vi "Operations Monitor.vi"() -> ()   [LabVIEW 2016, in "Top Level.lvlib"]
doc: "This VI is part of the Top Level library of VIs that are opened upon startup. Vacuum pressures are read via serial connections between the vacuum gauge controller and the nearest cRIO. At the cRIO, a Real-Time VI puts the pressures into shared variables which are displayed here. \n\nThe individual cRIOs are pinged to check network connections and cRIO resources are from shared variables. \n\nThe Omega CNi854 Controller/Monitor measures temperature of Cs Oven on ion source and is communicated with directly over TCP."
uses:
  Top Level.lvlib
  <vilib>/Utility/miscctls.llb/LVRowAndColumnTypeDef.ctl
  cRIO code/SCA/controls/GP307 cluster.ctl
panel:
  in  "Tab Control":T1(tab)
  out "LE Waist":string
  out "Tank Entrance":string
  out "Tank Exit":string
  out "Analyzer Image":string
  out "HE Waist/Analyzer Object":string
  out "Transmission":string
  out "R30 Switch Image":string
  out "R30 Detector":string
  out "R30 ESA":string
  in  "stop":bool
  out "date/time string":string
  out "Injector A Image":string
  out "Injector A Object":string
  out "Terminal Voltage":dbl format="%#_4g"
  out "R45 EXB":string
  out "R45 Switch Image":string
  out "R45 Waist":string
  out "SCA bellows":string
  out "SCA source":string
  in  "Ping Timeout (ms)":i32=100
  out "cRIO Status":i32(listbox)
  out "Oven Temperature":dbl(graph)
  out "Oven Temp (°C)":dbl
  in  "Omega VISA resource":refnum<visa-resource-name>="TCPIP0::192.168.1.173::2000::SOCKET"
  out "Omega Iteration":i32
  in  "byte count":u32=15
  in  "Wait (ms)":u32=500
  out "Read errors":i32
  out "Omega read buffer":string
  out "SV read error":errorcluster
  out "Terminal read error":errorcluster
  out "Ping error":errorcluster
  in  "Clear Ping Error":bool
  out "cRIO SV error":errorcluster
  in  "Clear SV Error":bool
  out "Omega T error":errorcluster
  # "VACUUM  PRESSURES"
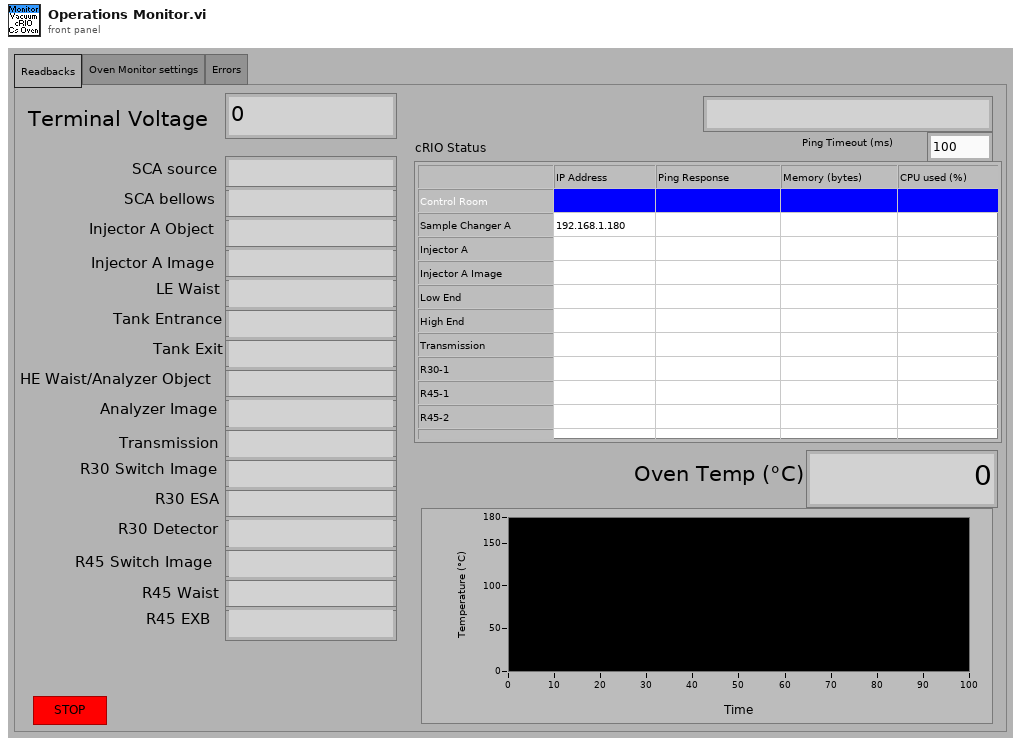
[diagram p1: front panel]
types:
  T1 = enum32{"Readbacks", "Oven Monitor settings", "Errors"}
  T2 = typedef "LVRowAndColumnTypeDef.ctl" = cluster{"Row":i32, "Column":i32}
  T3 = typedef "GP307 cluster.ctl" = cluster{"Ion gauge 1":string, "Convectron  Gauge 1 ":string, "Ion Gauge 2":string, "Convectrom Gauge 2":string}
  T4 = cluster{"Ion gauge 1":string, "Convectron  Gauge 1 ":string, "Ion Gauge 2":string, "Convectrom Gauge 2":string}
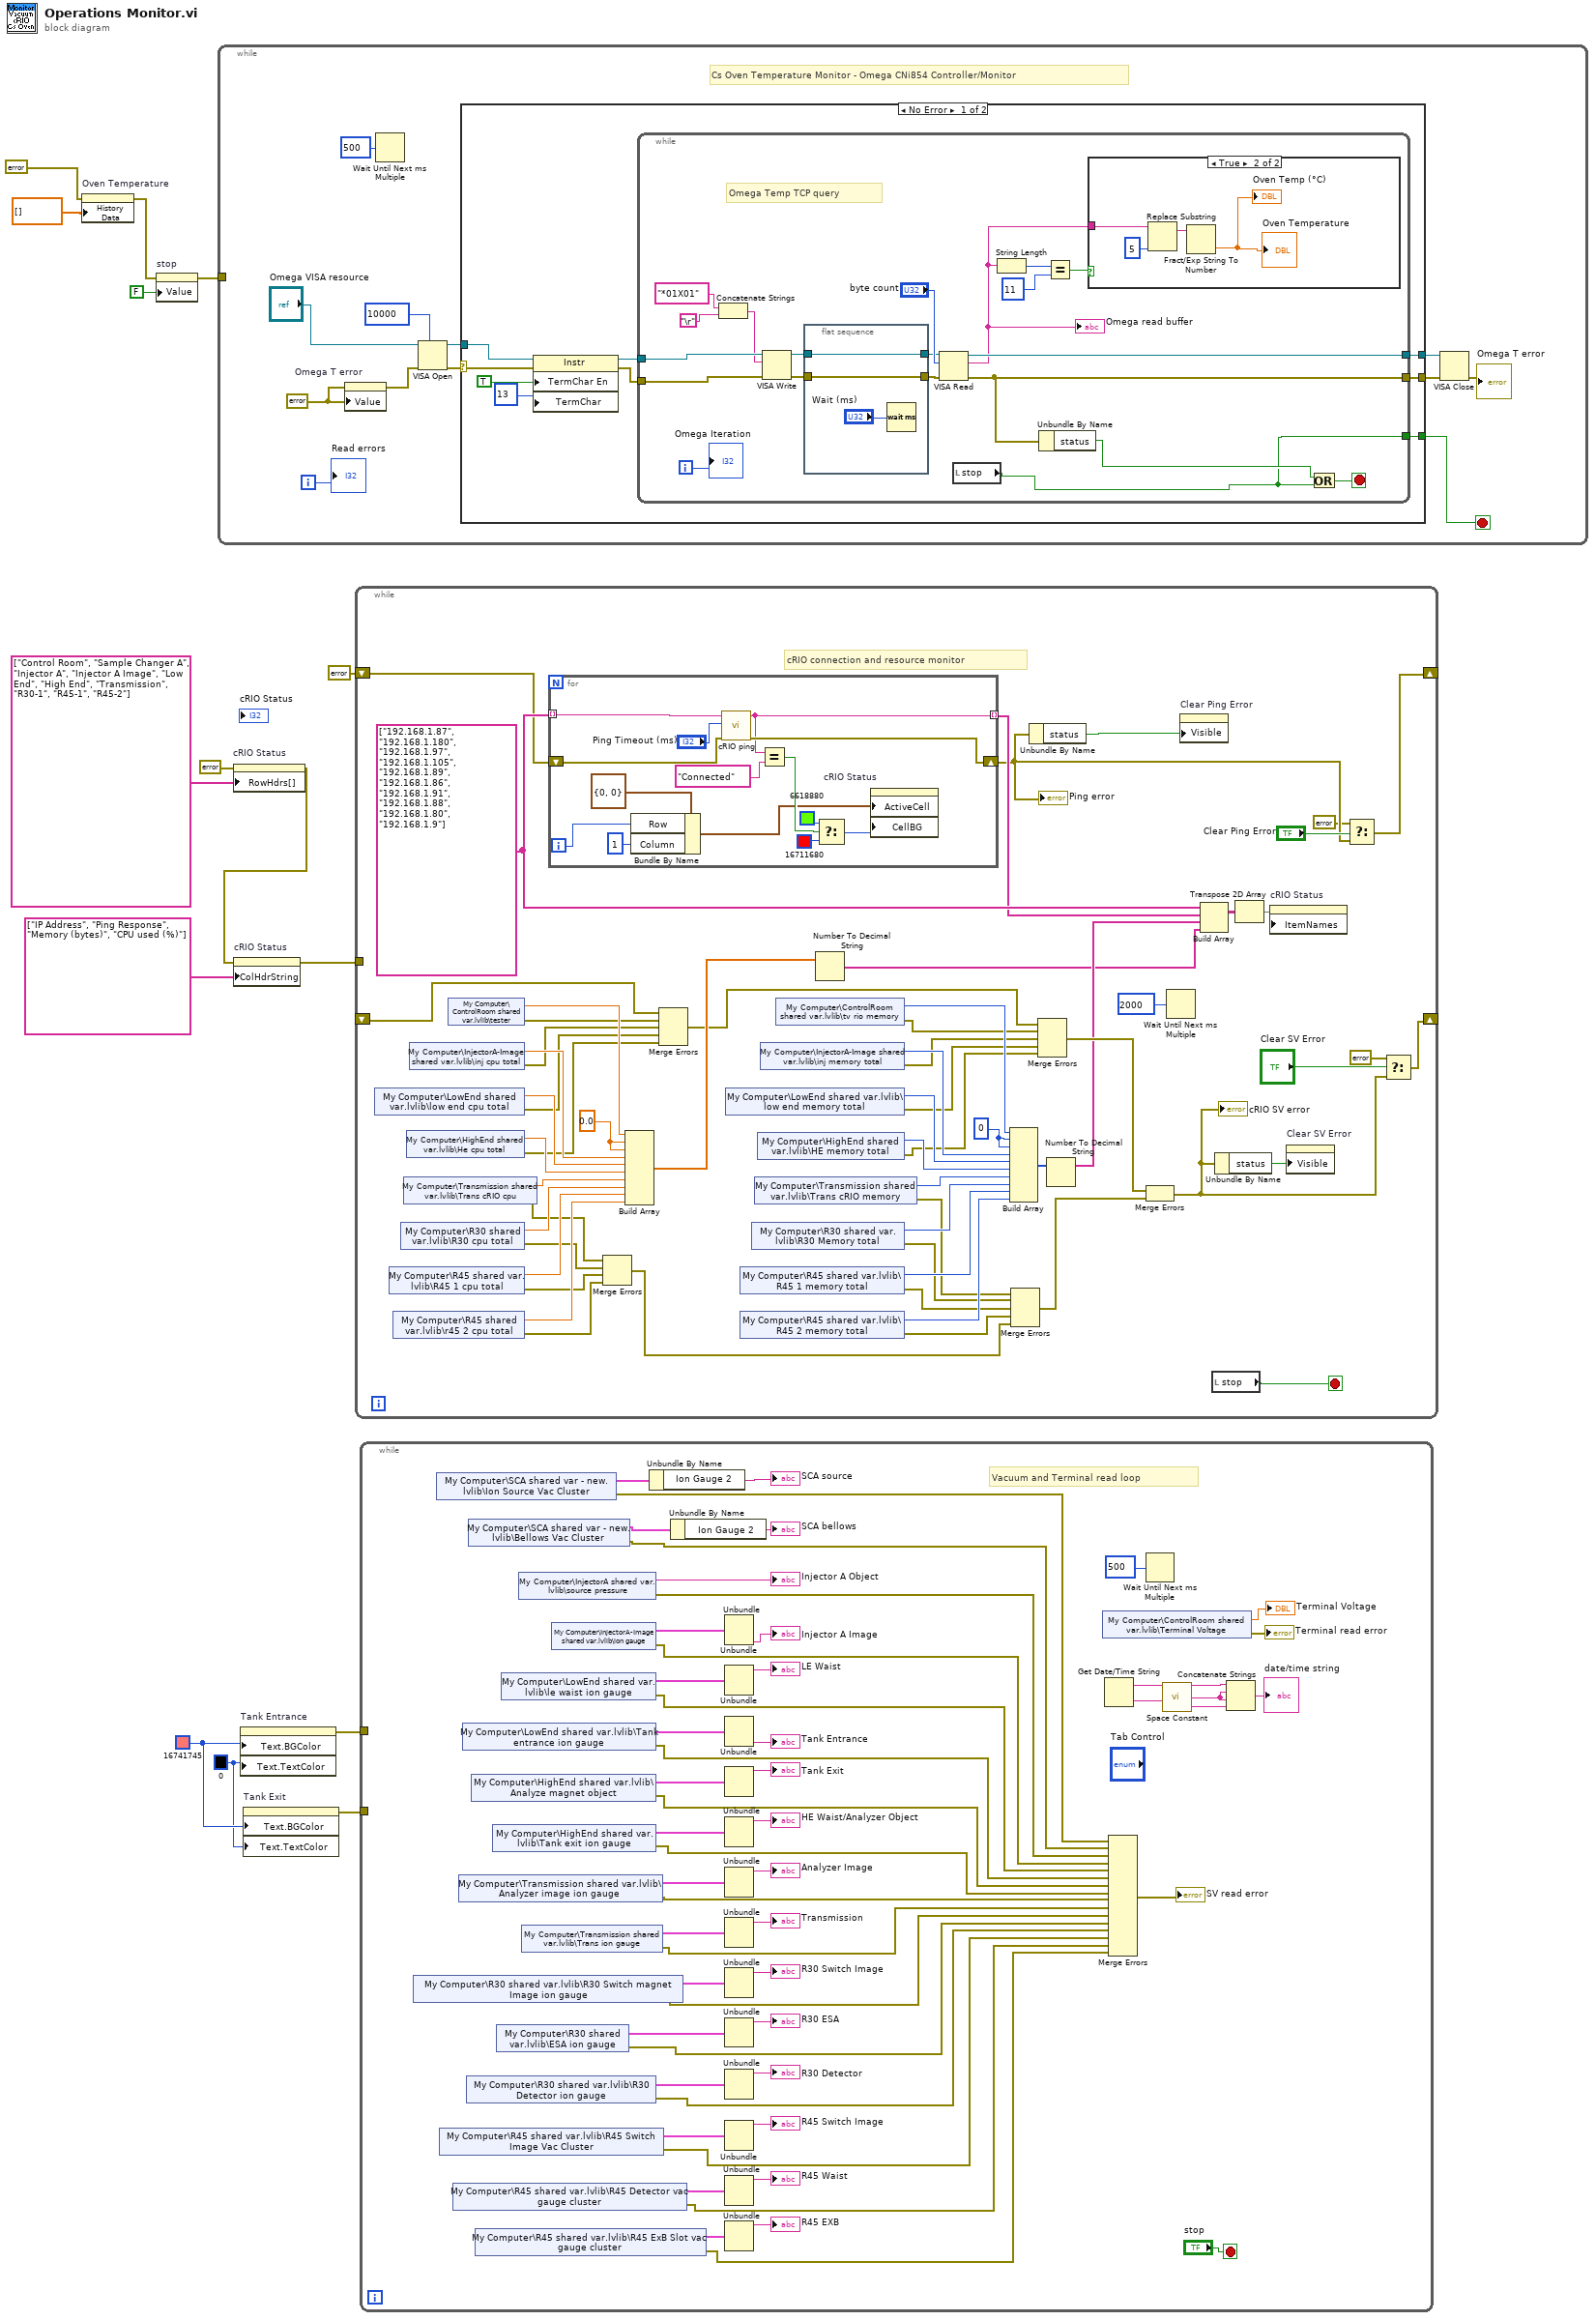
[diagram p0: block diagram]
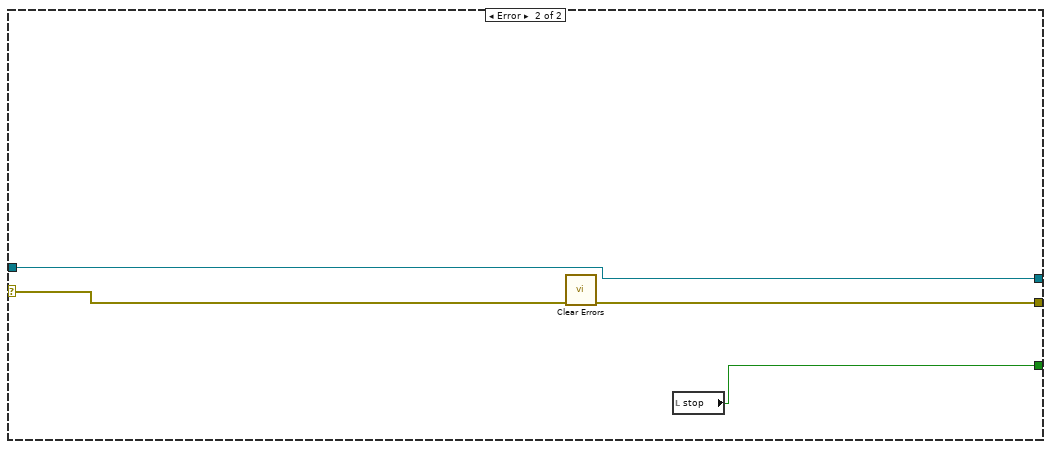
[diagram p3: hidden frame]
diagram:
  w1 = u32 0 ("Text.Text Colors:Text Color")
  w2 = u32 16741745 ("Text.Text Colors:BG Color")
  n1 = property on="Oven Temperature" class="WFChart (strict)"(error in=errorcluster {"status"=FALSE, "code"=0, "source"=""} ("error in (no error)"), "History Data"=dbl[] []) -> (error out=w6:errorcluster)  [unwired: 1 in, 1 out]
  n2 = property on="stop" class="Bool (strict)"(error in=w6, "Value"=FALSE ("stop")) -> (error out=w5:errorcluster)  [unwired: 1 in, 1 out]
  n3 = while {
    tunnel: w5 -> [_]
    i -> [w19]
    stop <- w20 stop-if-true
    w22 = errorcluster {"status"=FALSE, "code"=0, "source"=""} ("error in (no error)")
    # "Cs Oven Temperature Monitor - Omega CNi854 Controller/Monitor"
    # "Omega Temperature Monitor Loop"
    n4 = property on="Omega T error" class="Clust (strict)"(error in=w22, "Value"=w22) -> (error out=w23:errorcluster)  [unwired: 1 in, 1 out]
    n5 = Wait Until Next ms Multiple(millisecond multiple=u32 500) -> ()  [unwired: 1 out]
    n6 = VISA Open(timeout (0)=u32 10000 ("VISA Open timeout (0)"), error in (no error)=w23, VISA resource name="Omega VISA resource") -> (VISA resource name=w27:refnum<visa-resource-name>, error out=w18:errorcluster)  [unwired: 2 in]
    n7 = case shown="No Error" w18 {
      selector: w18 -> [w29 w66]
      tunnel: w27 -> [w34 w67]
      tunnel: [w36 w67] -> w26
      tunnel: [w35 w65] -> w25
      tunnel: [w30 w64] -> w20
      frame No Error {
        n8 = property class="Instr"(reference=w34, error in=w29, "TermChar En"=TRUE ("Message Based Settings:Termination Character Enable"), "TermChar"=u8 13 ("Message Based Settings:Termination Character")) -> (reference out=w33:refnum<visa-resource-name>, error out=w28:errorcluster)
        n9 = while {
          tunnel: w33 -> [w52]
          tunnel: [w56] -> w36
          tunnel: w28 -> [w47]
          tunnel: [w55] -> w35
          tunnel: [w37] -> w30
          i -> [w53]
          stop <- w54 stop-if-true
          # "Omega Temp TCP query"
          n10 = Concatenate Strings("*01X01" ("data in"), "\r") -> (w49:string)
          n11 = VISA Write(VISA resource name=w52, write buffer=w49, error in (no error)=w47) -> (VISA resource name out=w40:refnum<visa-resource-name>, error out=w42:errorcluster)  [unwired: 1 out]
          n12 = flat-sequence {
            tunnel: w42 -> [w59]
            tunnel: [w59] -> w41
            tunnel: w40 -> [w58]
            tunnel: [w58] -> w39
            frame #0 {
              n13 = Wait (ms)(milliseconds to wait="Wait (ms)") -> ()  [unwired: 1 out]
            }
          }
          n14 = VISA Read(VISA resource name=w39, byte count="byte count", error in (no error)=w41) -> (VISA resource name out=w56:refnum<visa-resource-name>, read buffer=w43:string, error out=w55:errorcluster)  [unwired: 1 out]
          "Omega read buffer" <- w43
          n15 = local read "stop"() -> (w37:bool)
          n16 = String Length(string=w43) -> (length=w46:i32)
          n17 = Unbundle By Name(w55) -> ("status"=w38:bool)
          n18 = Equal?(x=w46, y=11) -> (x = y?=w44:bool)
          n19 = case shown="True" w44 {
            tunnel: w43 -> [_ w60]
            frame False {
            }
            frame True {
              n20 = Replace Substring(2:5 ("length (len. of substring)"), 5:w60) -> (1:w61:string)  [unwired: 2 in, 1 out]
              n21 = Fract/Exp String To Number(string=w61) -> (number=→"Oven Temp (°C)" →"Oven Temperature":dbl)  [unwired: 3 in, 1 out]
            }
          }
          n22 = Or(x=w38, y=w37) -> (x .or. y?=w54:bool)
          "Omega Iteration" <- w53
        }
      }
      frame Error {
        n23 = call <vilib>:"Clear Errors.vi"("error in (no error)"=w66) -> ("error out"=w65:errorcluster)  [unwired: 5 in, 1 out]
        n24 = local read "stop"() -> (w64:bool)
      }
    }
    n25 = VISA Close(VISA resource name=w26, error in (no error)=w25) -> (error out=→"Omega T error":errorcluster)
    "Read errors" <- w19
  }
  n26 = property on="cRIO Status" class="MCListbox (strict)"(error in=errorcluster {"status"=FALSE, "code"=0, "source"=""} ("error out"), "RowHdrs[]"=string[] ["Control Room", "Sample Changer A", "Injector A", "Injector A Image", "Low End", "High End", "Transmission", "R30-1", "R45-1", "R45-2"]) -> (error out=w10:errorcluster)  [unwired: 1 in, 1 out]
  n27 = property on="cRIO Status" class="MCListbox (strict)"(error in=w10, "ColHdrString"=string[] ["IP Address", "Ping Response", "Memory (bytes)", "CPU used (%)"]) -> (error out=w13:errorcluster)  [unwired: 1 in, 1 out]
  n28 = property on="Tank Entrance" class="Str"("Text.BGColor"=w2, "Text.TextColor"=w1) -> (error out=w3:errorcluster)  [unwired: 2 in, 1 out]
  n29 = property on="Tank Exit" class="Str"("Text.BGColor"=w2, "Text.TextColor"=w1) -> (error out=w4:errorcluster)  [unwired: 2 in, 1 out]
  n30 = while {
    shift-right: [w72] -> _
    shift-left: _ -> [w97]
    shift-right: [w79] -> _
    shift-left: errorcluster {"status"=FALSE, "code"=0, "source"=""} ("Ping error out") -> [w104]
    tunnel: w13 -> [_]
    stop <- w70 stop-if-true
    w106 = string[] ["192.168.1.87", "192.168.1.180", "192.168.1.97", "192.168.1.105", "192.168.1.89", "192.168.1.86", "192.168.1.91", "192.168.1.88", "192.168.1.80", "192.168.1.9"]
    w107 = u32 0 ("element")
    w108 = 0.0 ("element")
    # "cRIO connection and resource monitor"
    n31 = shared-variable "My Computer\\LowEnd shared var.lvlib\\low end cpu total"() -> (w124:dbl, error out=w99:errorcluster)  [unwired: 1 in]
    n32 = shared-variable "My Computer\\R45 shared var.lvlib\\R45 1 cpu total"() -> (w120:dbl, error out=w96:errorcluster)  [unwired: 1 in]
    n33 = shared-variable "My Computer\\R45 shared var.lvlib\\r45 2 cpu total"() -> (w119:dbl, error out=w93:errorcluster)  [unwired: 1 in]
    n34 = shared-variable "My Computer\\R30 shared var.lvlib\\R30 cpu total"() -> (w121:dbl, error out=w95:errorcluster)  [unwired: 1 in]
    n35 = shared-variable "My Computer\\Transmission shared var.lvlib\\Trans cRIO cpu"() -> (w122:dbl, error out=w94:errorcluster)  [unwired: 1 in]
    n36 = shared-variable "My Computer\\HighEnd shared var.lvlib\\He cpu total"() -> (w123:dbl, error out=w98:errorcluster)  [unwired: 1 in]
    n37 = shared-variable "My Computer\\InjectorA-Image shared var.lvlib\\inj cpu total"() -> (w125:dbl, error out=w100:errorcluster)  [unwired: 1 in]
    n38 = shared-variable "My Computer\\ControlRoom shared var.lvlib\\tester"() -> (w126:dbl, error out=w101:errorcluster)  [unwired: 1 in]
    n39 = for {
      tunnel: w106 -> [w140] mode=indexing
      tunnel: [w137] -> w105 mode=indexing
      shift-right: [w138] -> w77
      shift-left: w104 -> [w139]
      i -> [w130]
      n40 = Bundle By Name(cluster=T2 {"Row"=0, "Column"=0} ("Active Cell:Active Cell"), "Row"=w130, "Column"=1) -> (w129:T2)
      n41 = call "cRIO ping.vi"("Error in"=w139, "Ping Timeout (ms)"="Ping Timeout (ms)", "IP Address"=w140) -> ("Ping error out"=w138:errorcluster, "Ping Response"=w137:string)  [unwired: 7 in]
      n42 = Equal?(x=w137, y="Connected" ("t")) -> (x = y?=w134:bool)
      n43 = Select(t=u32 6618880, s=w134, f=u32 16711680) -> (s? t:f=w135:u32)
      n44 = property on="cRIO Status" class="MCListbox (strict)"("ActiveCell"=w129, "CellBG"=w135) -> ()  [unwired: 2 in, 2 out]
    }
    "Ping error" <- w77
    n45 = Merge Errors(w94, w95, w96, w93) -> (w82:errorcluster)
    n46 = Build Array(w126, w108, w108, w125, w124, w123, w122, w121, w120, w119) -> (w109:dbl[])
    n47 = Merge Errors(w97, w101, w100, w99, w98) -> (w92:errorcluster)
    n48 = shared-variable "My Computer\\LowEnd shared var.lvlib\\low end memory total"() -> (w112:u32, error out=w89:errorcluster)  [unwired: 1 in]
    n49 = shared-variable "My Computer\\R45 shared var.lvlib\\R45 1 memory total"() -> (w116:u32, error out=w86:errorcluster)  [unwired: 1 in]
    n50 = shared-variable "My Computer\\R45 shared var.lvlib\\R45 2 memory total"() -> (w117:u32, error out=w87:errorcluster)  [unwired: 1 in]
    n51 = shared-variable "My Computer\\R30 shared var.lvlib\\R30 Memory total"() -> (w115:u32, error out=w85:errorcluster)  [unwired: 1 in]
    n52 = shared-variable "My Computer\\Transmission shared var.lvlib\\Trans cRIO memory"() -> (w114:u32, error out=w84:errorcluster)  [unwired: 1 in]
    n53 = shared-variable "My Computer\\HighEnd shared var.lvlib\\HE memory total"() -> (w111:u32, error out=w88:errorcluster)  [unwired: 1 in]
    n54 = shared-variable "My Computer\\InjectorA-Image shared var.lvlib\\inj memory total"() -> (w113:u32, error out=w90:errorcluster)  [unwired: 1 in]
    n55 = shared-variable "My Computer\\ControlRoom shared var.lvlib\\tv rio memory"() -> (w118:u32, error out=w91:errorcluster)  [unwired: 1 in]
    n56 = Number To Decimal String(number=w109) -> (decimal integer string=w68:string[])  [unwired: 1 in]
    n57 = Build Array(w118, w107, w107, w113, w112, w111, w114, w115, w116, w117) -> (w110:u32[])
    n58 = Merge Errors(w84, w85, w86, w87, w82) -> (w83:errorcluster)
    n59 = Unbundle By Name(w77) -> ("status"=w80:bool)
    n60 = Merge Errors(w92, w91, w90, w89, w88) -> (w81:errorcluster)
    n61 = Number To Decimal String(number=w110) -> (decimal integer string=w69:string[])  [unwired: 1 in]
    n62 = Merge Errors(w81, w83) -> (w71:errorcluster)
    "cRIO SV error" <- w71
    n63 = Wait Until Next ms Multiple(millisecond multiple=u32 2000) -> ()  [unwired: 1 out]
    n64 = property on="Clear Ping Error" class="Bool"("Visible"=w80) -> ()  [unwired: 2 in, 2 out]
    n65 = Build Array(w106, w105, w69, w68) -> (w103:string[][])
    n66 = local read "stop"() -> (w70:bool)
    n67 = Unbundle By Name(w71) -> ("status"=w75:bool)
    n68 = Transpose 2D Array(2D array=w103) -> (transposed array=w102:string[][])
    n69 = property on="cRIO Status" class="MCListbox (strict)"("ItemNames"=w102) -> ()  [unwired: 2 in, 2 out]
    n70 = property on="Clear SV Error" class="Bool"("Visible"=w75) -> ()  [unwired: 2 in, 2 out]
    n71 = Select(t=errorcluster {"status"=FALSE, "code"=0, "source"=""}, s="Clear Ping Error", f=w77) -> (s? t:f=w79:errorcluster)
    n72 = Select(t=errorcluster {"status"=FALSE, "code"=0, "source"=""}, s="Clear SV Error", f=w71) -> (s? t:f=w72:errorcluster)
  }
  n73 = while {
    tunnel: w4 -> [_]
    tunnel: w3 -> [_]
    stop <- "stop" stop-if-true
    # "Vacuum and Terminal read loop"
    n74 = shared-variable "My Computer\\R30 shared var.lvlib\\R30 Switch magnet Image ion gauge"() -> (w183:cluster{string, string, string, string}, error out=w155:errorcluster)  [unwired: 1 in]
    n75 = shared-variable "My Computer\\SCA shared var - new.lvlib\\Ion Source Vac Cluster"() -> (w146:T3, error out=w147:errorcluster)  [unwired: 1 in]
    n76 = shared-variable "My Computer\\R45 shared var.lvlib\\R45 Switch Image Vac Cluster"() -> (w178:T4, error out=w152:errorcluster)  [unwired: 1 in]
    n77 = shared-variable "My Computer\\R45 shared var.lvlib\\R45 Detector vac gauge cluster"() -> (w177:T4, error out=w151:errorcluster)  [unwired: 1 in]
    n78 = shared-variable "My Computer\\Transmission shared var.lvlib\\Analyzer image ion gauge"() -> (w185:T4, error out=w157:errorcluster)  [unwired: 1 in]
    n79 = shared-variable "My Computer\\LowEnd shared var.lvlib\\Tank entrance ion gauge"() -> (w194:cluster{string, string, string, string}, error out=w160:errorcluster)  [unwired: 1 in]
    n80 = shared-variable "My Computer\\R30 shared var.lvlib\\R30 Detector ion gauge"() -> (w182:cluster{string, string, string, string}, error out=w153:errorcluster)  [unwired: 1 in]
    n81 = shared-variable "My Computer\\SCA shared var - new.lvlib\\Bellows Vac Cluster"() -> (w143:T3, error out=w144:errorcluster)  [unwired: 1 in]
    n82 = shared-variable "My Computer\\HighEnd shared var.lvlib\\Analyze magnet object"() -> (w193:cluster{string, string, string, string}, error out=w159:errorcluster)  [unwired: 1 in]
    n83 = shared-variable "My Computer\\R45 shared var.lvlib\\R45 ExB Slot vac gauge cluster"() -> (w179:T4, error out=w150:errorcluster)  [unwired: 1 in]
    n84 = shared-variable "My Computer\\HighEnd shared var.lvlib\\Tank exit ion gauge"() -> (w192:cluster{string, string, string, string}, error out=w158:errorcluster)  [unwired: 1 in]
    n85 = shared-variable "My Computer\\R30 shared var.lvlib\\ESA ion gauge"() -> (w181:cluster{string, string, string, string}, error out=w154:errorcluster)  [unwired: 1 in]
    n86 = shared-variable "My Computer\\LowEnd shared var.lvlib\\le waist ion gauge"() -> (w195:cluster{string, string, string, string}, error out=w161:errorcluster)  [unwired: 1 in]
    n87 = shared-variable "My Computer\\InjectorA shared var.lvlib\\source pressure"() -> (→"Injector A Object":string, error out=w163:errorcluster)  [unwired: 1 in]
    n88 = shared-variable "My Computer\\Transmission shared var.lvlib\\Trans ion gauge"() -> (w184:T4, error out=w156:errorcluster)  [unwired: 1 in]
    n89 = shared-variable "My Computer\\InjectorA-Image shared var.lvlib\\ion gauge"() -> (w191:cluster{string, string, string, string}, error out=w162:errorcluster)  [unwired: 1 in]
    n90 = Unbundle By Name(w146) -> ("Ion Gauge 2"=→"SCA source":string)
    n91 = Unbundle By Name(w143) -> ("Ion Gauge 2"=→"SCA bellows":string)
    n92 = Unbundle(w191) -> (→"Injector A Image":string)  [unwired: 3 out]
    n93 = Unbundle(w195) -> (→"LE Waist":string)  [unwired: 3 out]
    n94 = Unbundle(w194) -> (→"Tank Entrance":string)  [unwired: 3 out]
    n95 = Unbundle(w193) -> (→"Tank Exit":string)  [unwired: 3 out]
    n96 = Unbundle(w192) -> (→"HE Waist/Analyzer Object":string)  [unwired: 3 out]
    n97 = Unbundle(w185) -> ("Ion gauge 1"=→"Analyzer Image":string)  [unwired: 3 out]
    n98 = Unbundle(w184) -> ("Ion gauge 1"=→"Transmission":string)  [unwired: 3 out]
    n99 = Unbundle(w183) -> (→"R30 Switch Image":string)  [unwired: 3 out]
    n100 = Unbundle(w181) -> (→"R30 ESA":string)  [unwired: 3 out]
    n101 = Unbundle(w182) -> (→"R30 Detector":string)  [unwired: 3 out]
    n102 = Unbundle(w178) -> ("Ion gauge 1"=→"R45 Switch Image":string)  [unwired: 3 out]
    n103 = Unbundle(w177) -> ("Ion gauge 1"=→"R45 Waist":string)  [unwired: 3 out]
    n104 = Unbundle(w179) -> ("Ion gauge 1"=→"R45 EXB":string)  [unwired: 3 out]
    n105 = shared-variable "My Computer\\ControlRoom shared var.lvlib\\Terminal Voltage"() -> (→"Terminal Voltage":dbl, error out=→"Terminal read error":errorcluster)  [unwired: 1 in]
    n106 = Get Date/Time String() -> (date string=w189:string, time string=w186:string)  [unwired: 3 in]
    n107 = Merge Errors(w147, w144, w163, w162, w161, w160, w159, w158, w157, w156, w155, w154, w153, w152, w151, w150) -> (→"SV read error":errorcluster)
    n108 = Wait Until Next ms Multiple(millisecond multiple=u32 500) -> ()  [unwired: 1 out]
    n109 = call <vilib>:"Space Constant.vi"() -> ("String"=w187:string)
    n110 = Concatenate Strings(w189, w187, w187, w186) -> (→"date/time string":string)
  }
